vi "Resistance cal.vi"() -> ()   [LabVIEW 2013]
panel:
  out "Tolerance":string
  in  "Colour  5":u16(ring) items=["Brown", "Red", "Yellow", "Green", "Blue", "Violet", "Gray", "Gold", "silver", "No colour"]
  in  "colour 4":u16(ring) items=["Black", "Brown", "Red", "Orange", "Yellow", "Green", "Blue", "Violet", "Gray", "White", "Gold", "silver"]
  in  "Colour 3":u16(ring) items=["Black", "Brown", "Red", "Orange", "Yellow", "Green", "Blue", "Violet", "Gray", "White", "Gold", "silver"]
  in  "Colour 2":u16(ring) items=["Black", "Brown", "Red", "Orange", "Yellow", "Green", "Blue", "Violet", "Gray", "White", "Gold", "silver"]
  in  "Colour 1":T1(ring)
  in  "?":bool
  out "Ohms":u64
  # "Resisitance Calculation"
  # "4 Colour"
  # "%"
  # "3 Colour"
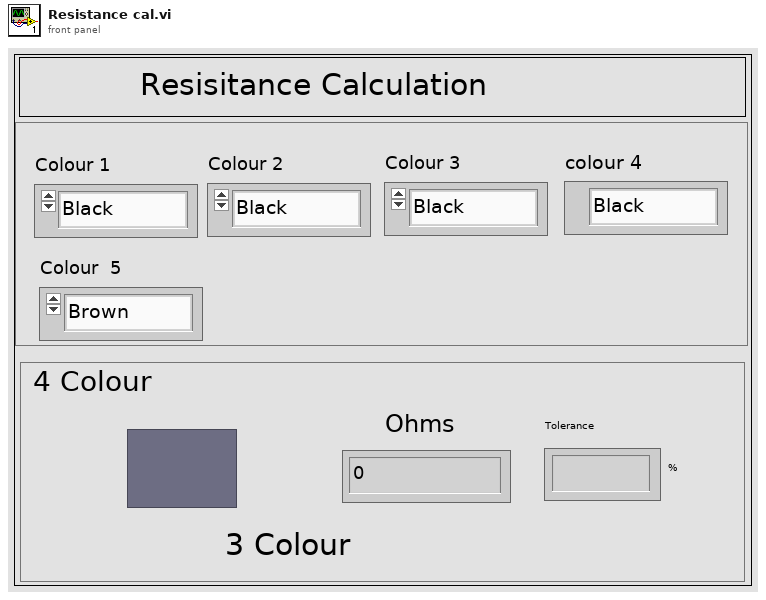
[diagram p1: front panel]
types:
  T1 = enum16{"Black", "Brown", "Red", "Orange", "Yellow", "Green", "Blue", "Violet", "Gray", "White", "Gold", "silver"}
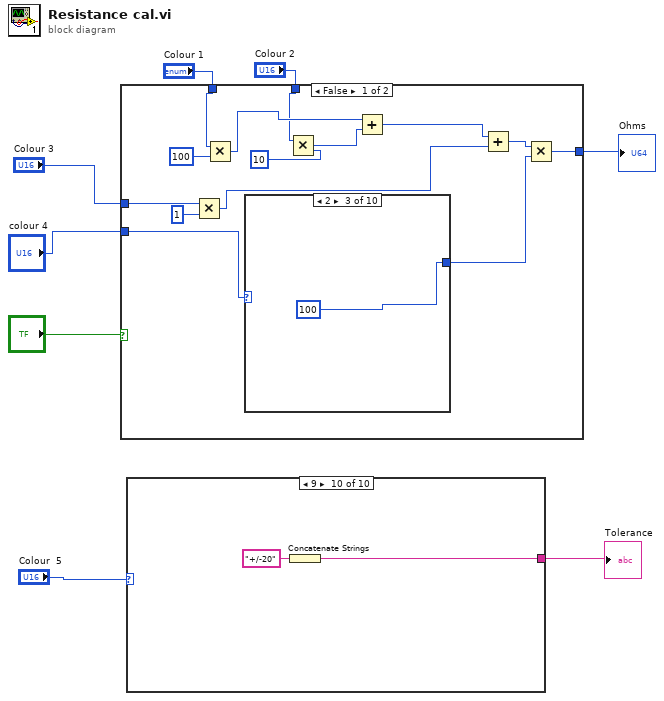
[diagram p0: block diagram]
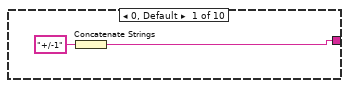
[diagram p2: hidden frame]
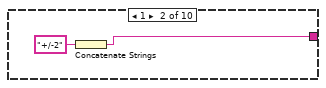
[diagram p3: hidden frame]
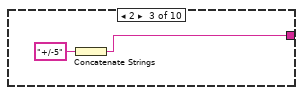
[diagram p4: hidden frame]
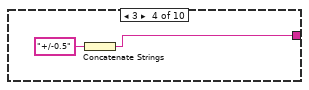
[diagram p5: hidden frame]
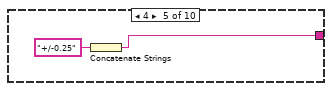
[diagram p6: hidden frame]
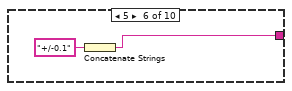
[diagram p7: hidden frame]
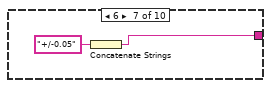
[diagram p8: hidden frame]
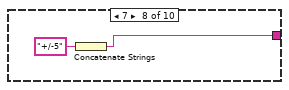
[diagram p9: hidden frame]
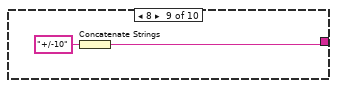
[diagram p10: hidden frame]
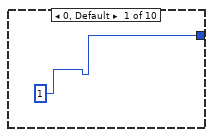
[diagram p11: hidden frame]
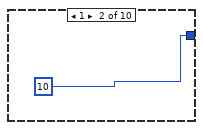
[diagram p12: hidden frame]
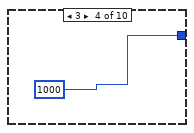
[diagram p13: hidden frame]
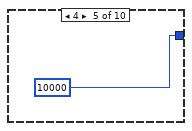
[diagram p14: hidden frame]
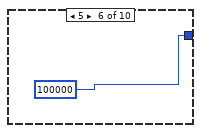
[diagram p15: hidden frame]
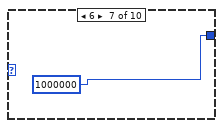
[diagram p16: hidden frame]
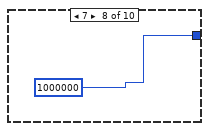
[diagram p17: hidden frame]
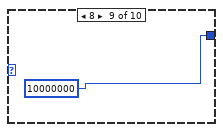
[diagram p18: hidden frame]
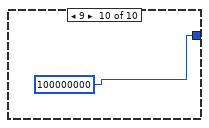
[diagram p19: hidden frame]
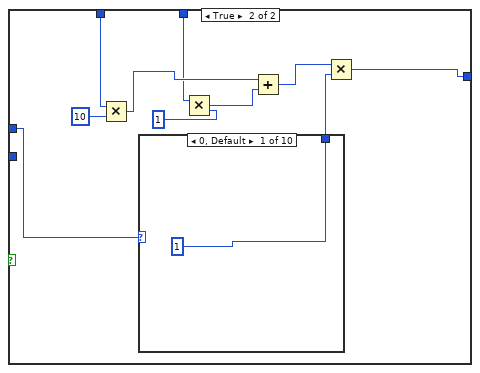
[diagram p20: hidden frame]
diagram:
  n1 = case shown="False" "?" {
    tunnel: "Colour 1" -> [w18 w37]
    tunnel: "Colour 2" -> [w17 w36]
    tunnel: [w11 w35] -> w6
    tunnel: "colour 4" -> [w10 _]
    tunnel: "Colour 3" -> [w9 w33]
    frame False {
      n2 = Multiply(x=w9, y=u16 1) -> (x*y=w15:u16)
      n3 = Multiply(x=w18, y=u16 100) -> (x*y=w20:u16)
      n4 = case shown="2" w10 {
        tunnel: [u16 1 ("y") u16 10 ("y") u16 100 ("y") u16 1000 ("y") u16 10000 ("y") u64 100000 ("y") u64 1000000 ("y") u64 1000000 ("y") u64 10000000 ("y") u64 100000000 ("y")] -> w12
        frame 0, Default {
        }
        frame 1 {
        }
        frame 2 {
        }
        frame 3 {
        }
        frame 4 {
        }
        frame 5 {
        }
        frame 6 {
        }
        frame 7 {
        }
        frame 8 {
        }
        frame 9 {
        }
      }
      n5 = Multiply(x=w17, y=u16 10) -> (x*y=w19:u16)
      n6 = Add(x=w20, y=w19) -> (x+y=w14:u16)
      n7 = Add(x=w14, y=w15) -> (x+y=w13:u16)
      n8 = Multiply(x=w13, y=w12) -> (x*y=w11:u64)
    }
    frame True {
      n9 = Multiply(x=w37, y=u16 10) -> (x*y=w40:u16)
      n10 = case shown="0, Default" w33 {
        tunnel: [u16 1 ("y") u16 10 ("y") u16 100 ("y") u16 1000 ("y") u16 10000 ("y") u64 100000 ("y") u64 1000000 ("y") u64 1000000 ("y") u64 10000000 ("y") u64 100000000 ("y")] -> w34
        frame 0, Default {
        }
        frame 1 {
        }
        frame 2 {
        }
        frame 3 {
        }
        frame 4 {
        }
        frame 5 {
        }
        frame 6 {
        }
        frame 7 {
        }
        frame 8 {
        }
        frame 9 {
        }
      }
      n11 = Multiply(x=w36, y=u16 1) -> (x*y=w39:u16)
      n12 = Add(x=w40, y=w39) -> (x+y=w38:u16)
      n13 = Multiply(x=w38, y=w34) -> (x*y=w35:u64)
    }
  }
  "Ohms" <- w6
  n14 = case shown="9" "Colour  5" {
    tunnel: [w53 w55 w57 w59 w61 w63 w65 w67 w69 w71] -> w1
    frame 0, Default {
      n15 = Concatenate Strings("+/-1" ("string")) -> (w53:string)
    }
    frame 1 {
      n16 = Concatenate Strings("+/-2" ("string")) -> (w55:string)
    }
    frame 2 {
      n17 = Concatenate Strings("+/-5" ("string")) -> (w57:string)
    }
    frame 3 {
      n18 = Concatenate Strings("+/-0.5" ("string")) -> (w59:string)
    }
    frame 4 {
      n19 = Concatenate Strings("+/-0.25" ("string")) -> (w61:string)
    }
    frame 5 {
      n20 = Concatenate Strings("+/-0.1" ("string")) -> (w63:string)
    }
    frame 6 {
      n21 = Concatenate Strings("+/-0.05" ("string")) -> (w65:string)
    }
    frame 7 {
      n22 = Concatenate Strings("+/-5" ("string")) -> (w67:string)
    }
    frame 8 {
      n23 = Concatenate Strings("+/-10" ("string")) -> (w69:string)
    }
    frame 9 {
      n24 = Concatenate Strings("+/-20" ("string")) -> (w71:string)
    }
  }
  "Tolerance" <- w1
